vi "LoadSettingGeneral.vi"(8 "error in (no error)":errorcluster, 11 "Gviewer in":refnum<class "Gviewer.lvclass">) -> (0 "error out":errorcluster, 2 "SettingsGeneral":T1, 3 "Gviewer out":refnum<class "Gviewer.lvclass">)   [LabVIEW 2020, in "Sgraph_lib_V1.lvlib" / "Gviewer.lvclass"]
doc: "Get General Settings\n(applicable for all instances of Gviewer simultaneously)"
uses:
  Gviewer.lvclass
  controls/SettingsGeneral.ctl
  Gviewer.lvclass/Gviewer.ctl
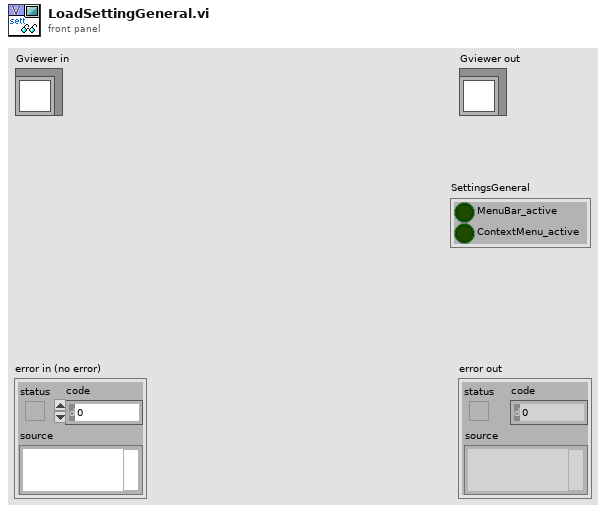
[diagram p1: front panel]
types:
  T1 = typedef "Sgraph_lib_V1.lvlib/Gviewer.lvclass/SettingsGeneral.ctl" = cluster{"MenuBar_active":bool, "ContextMenu_active":bool}
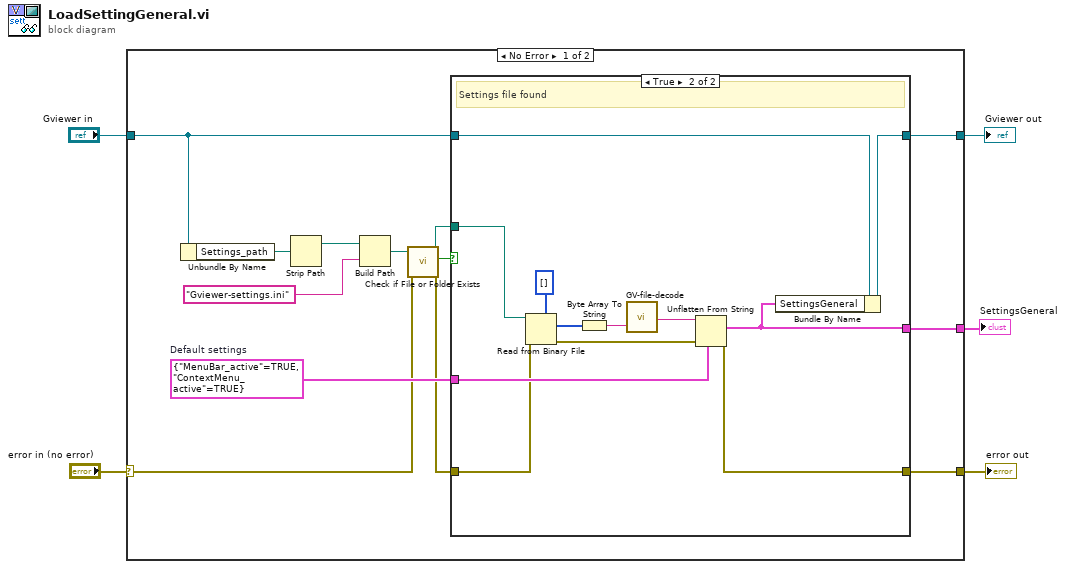
[diagram p0: block diagram]
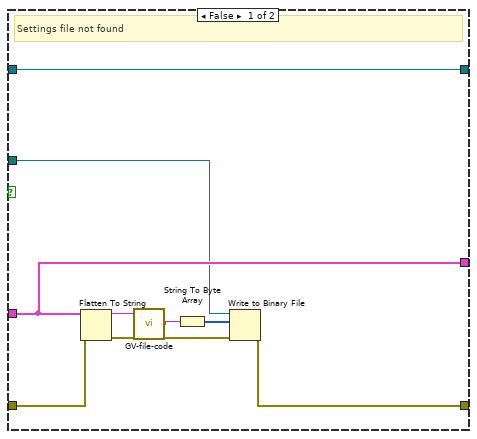
[diagram p2: hidden frame]
diagram:
  n1 = case shown="No Error" "error in (no error)" {
    selector: "error in (no error)" -> [w7 w41]
    tunnel: [w11 w41] -> w4
    tunnel: [w12 w40] -> w2
    tunnel: "Gviewer in" -> [w13 w40]
    tunnel: [w9 _] -> w1
    frame No Error {
      w10 = T1 {"MenuBar_active"=TRUE, "ContextMenu_active"=TRUE}  # Default settings
      n2 = Unbundle By Name(w13) -> ("Settings_path"=w18:path)
      n3 = Strip Path(path=w18) -> (stripped path=w17:path)  [unwired: 1 out]
      n4 = Build Path(base path=w17, name or relative path="Gviewer-settings.ini") -> (appended path=w15:path)
      n5 = call <vilib>:"Check if File or Folder Exists.vi"("error in (no error)"=w7, "path"=w15) -> ("error out"=w6:errorcluster, "file or folder exists?"=w14:bool, "dup path"=w8:path)  [unwired: 7 in]
      n6 = case shown="True" w14 {
        tunnel: w13 -> [w27 w30]
        tunnel: w6 -> [w21 w33]
        tunnel: [w27 w31] -> w12
        tunnel: [w22 w34] -> w11
        tunnel: w10 -> [w25 w36]
        tunnel: [w25 w32] -> w9
        tunnel: w8 -> [w24 w39]
        frame False {
          # "Settings file not found"
          n7 = Flatten To String(anything=w25, error in (no error)=w21) -> (data string=w26:string, error out=w23:errorcluster)  [unwired: 2 in, 1 out]
          n8 = call "GV-file-code.vi"("string input"=w26) -> ("string output"=w20:string)  [unwired: 1 in]
          n9 = String To Byte Array(string=w20) -> (unsigned byte array=w19:u8[])
          n10 = Write to Binary File(file (use dialog)=w24, data=w19, error in=w23) -> (error out=w22:errorcluster)  [unwired: 3 in, 2 out]
        }
        frame True {
          # "Settings file found"
          n11 = Read from Binary File(5:u8[] [] ("unsigned byte array"), 8:w33, 11:w39) -> (0:w35:errorcluster, 2:w38:u8[])  [unwired: 3 in, 2 out]
          n12 = Byte Array To String(unsigned byte array=w38) -> (string=w28:string)
          n13 = call "GV-file-decode.vi"("string input"=w28) -> ("string output"=w37:string)  [unwired: 1 in]
          n14 = Unflatten From String(type=w36, binary string=w37, error in (no error)=w35) -> (value=w32:T1, error out=w34:errorcluster)  [unwired: 2 in, 1 out]
          n15 = Bundle By Name(cluster=w30, "SettingsGeneral"=w32) -> (w31:refnum<class "Gviewer.lvclass">)
        }
      }
    }
    frame Error {
    }
  }
  "error out" <- w4
  "Gviewer out" <- w2
  "SettingsGeneral" <- w1
